vi "LEDC Control Loop 1931 Init.vi"(0 "LEDAD Port":refnum<visa-resource-name>="COM9", 1 "Wavelength":string="1550", 5 "Light Meter Port":refnum<visa-resource-name>="COM3", 9 "Illumination Cal Factor":dbl=0.444212 format="%#.6f", 11 "error in (no error)":errorcluster, 12 "Unit":u16(ring) items=["nW/cm^2", "pW/cm^2"]) -> (3 "In Progress":bool, 4 "LEDAD Port out":refnum<visa-resource-name>, 6 "Light Meter Port out":refnum<visa-resource-name>, 8 "WL>800":bool, 10 "Max Illum":dbl format="%#_4g", 14 "Done":bool, 15 "error out":errorcluster)   [LabVIEW 2010]
panel:
  # "nm"
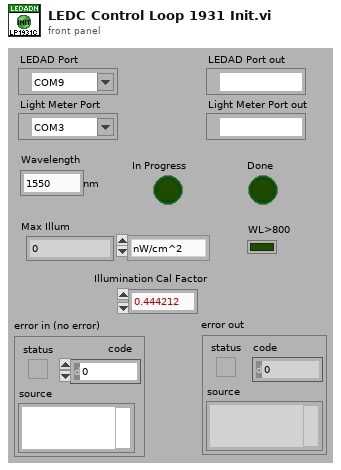
[diagram p1: front panel]
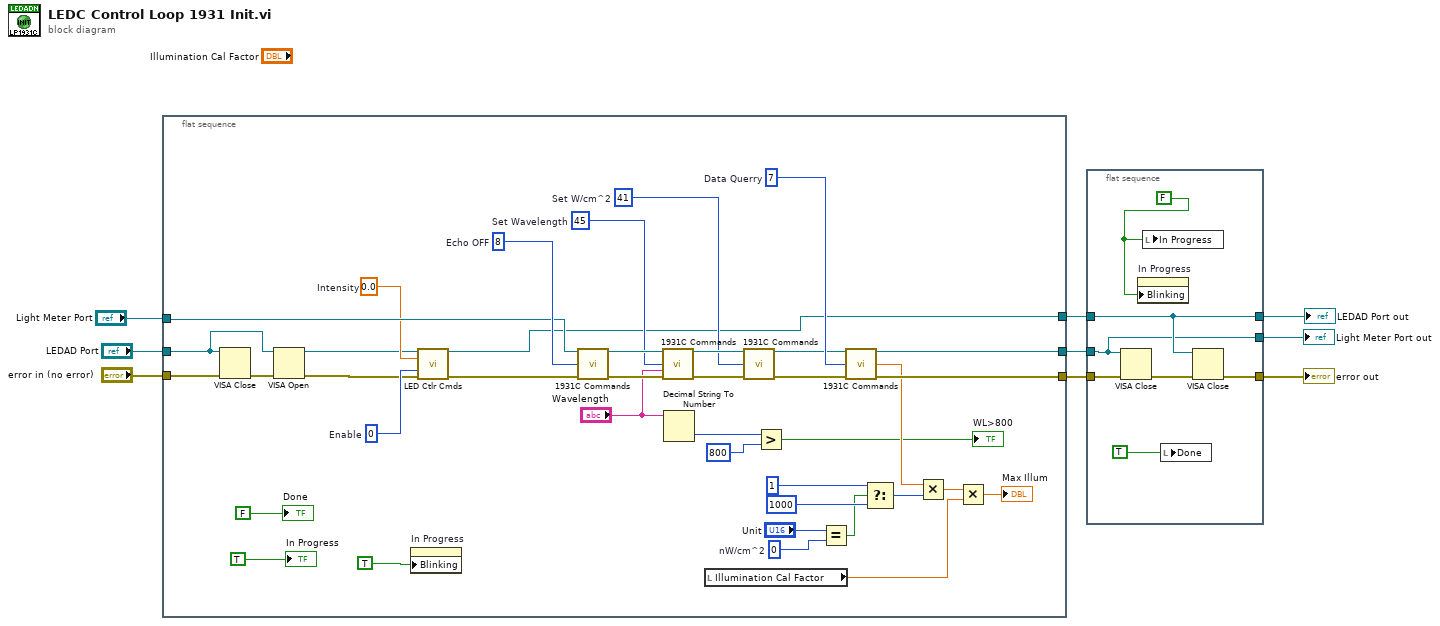
[diagram p0: block diagram]
diagram:
  n1 = flat-sequence {
    tunnel: "error in (no error)" -> [w48]
    tunnel: "LEDAD Port" -> [w46]
    tunnel: "Light Meter Port" -> [w22]
    tunnel: [w40] -> w2
    tunnel: [w39] -> w3
    tunnel: [w11] -> w1
    frame #0 {
      w27 = 41  # Set W/cm^2
      w33 = 0  # nW/cm^2
      w41 = 7  # Data Querry
      w42 = 45  # Set Wavelength
      w45 = 8  # Echo OFF
      w14 = u8 0  # Enable
      w15 = 0.0  # Intensity
      n2 = VISA Close(VISA resource name=w46, error in (no error)=w48) -> (error out=w47:errorcluster)
      n3 = VISA Open(error in (no error)=w47, VISA resource name=w46) -> (VISA resource name=w13:refnum<visa-resource-name>, error out=w12:errorcluster)  [unwired: 3 in]
      n4 = property on="In Progress" class="Bool (strict)"("Blinking"=TRUE) -> ()  [unwired: 2 in, 2 out]
      n5 = call "LED Ctlr Cmds.vi"("VISA session"=w13, "Intensity"=w15, "Enable"=w14, "error in (no error)"=w12) -> ("VISA session out"=w11:refnum<visa-resource-name>, "error out"=w10:errorcluster)  [unwired: 7 in, 3 out]
      n6 = call "1931C Commands.vi"("Instrument Resource Name"=w22, "Command"=w45, "error in (no error)"=w10) -> ("VISA resource name out"=w43:refnum<visa-resource-name>, "error out"=w44:errorcluster)  [unwired: 8 in, 3 out]
      n7 = call "1931C Commands.vi"("Instrument Resource Name"=w43, "Command"=w42, "Wavelength"="Wavelength", "error in (no error)"=w44) -> ("VISA resource name out"=w28:refnum<visa-resource-name>, "error out"=w29:errorcluster)  [unwired: 7 in, 3 out]
      n8 = Decimal String To Number(string="Wavelength") -> (number=w24:i32)  [unwired: 2 in, 1 out]
      n9 = local read "Illumination Cal Factor"() -> (w17:dbl)
      n10 = call "1931C Commands.vi"("Instrument Resource Name"=w28, "Command"=w27, "error in (no error)"=w29) -> ("VISA resource name out"=w21:refnum<visa-resource-name>, "error out"=w19:errorcluster)  [unwired: 8 in, 3 out]
      n11 = Greater?(x=w24, y=800) -> (0:→"WL>800":bool)
      n12 = Equal?(x="Unit", y=w33) -> (x = y?=w32:bool)
      n13 = call "1931C Commands.vi"("Instrument Resource Name"=w21, "Command"=w41, "error in (no error)"=w19) -> ("VISA resource name out"=w40:refnum<visa-resource-name>, "LM Response"=w31:dbl, "error out"=w39:errorcluster)  [unwired: 8 in, 2 out]
      n14 = Select(t=1, s=w32, f=1000) -> (s? t:f=w26:i32)
      n15 = Multiply(x=w31, y=w26) -> (x*y=w18:dbl)
      n16 = Multiply(x=w18, y=w17) -> (x*y=→"Max Illum":dbl)
      "Done" <- FALSE
      "In Progress" <- TRUE
    }
  }
  n17 = flat-sequence {
    tunnel: w2 -> [w51]
    tunnel: w3 -> [w53]
    tunnel: [w52] -> w4
    tunnel: w1 -> [w52]
    tunnel: [w51] -> w5
    tunnel: [w49] -> w6
    frame #0 {
      w55 = FALSE
      n18 = VISA Close(VISA resource name=w51, error in (no error)=w53) -> (error out=w50:errorcluster)
      n19 = property on="In Progress" class="Bool (strict)"("Blinking"=w55) -> ()  [unwired: 2 in, 2 out]
      n20 = local write "In Progress"(w55) -> ()
      n21 = local write "Done"(TRUE) -> ()
      n22 = VISA Close(VISA resource name=w52, error in (no error)=w50) -> (error out=w49:errorcluster)
    }
  }
  "LEDAD Port out" <- w4
  "Light Meter Port out" <- w5
  "error out" <- w6
